vi "Log Error.vi"(10 "Log Packet":T1, 11 "Application Log in":refnum<class "Application Logger.lvclass">) -> (0 "error out":errorcluster, 3 "Application Log out":refnum<class "Application Logger.lvclass">)   [LabVIEW 2017, in "Composed Log.lvlib" / "Application Logger.lvclass"]
uses:
  <vilib>/gpm_packages/@cs/event-logger/Source/Composed Log/Application Logger/Application Logger.lvclass
  <vilib>/gpm_packages/@cs/event-logger/Source/Composed Log/Types/Log Packet.ctl
  <vilib>/gpm_packages/@cs/event-logger/Source/Composed Log/Types/Log Level.ctl
  <vilib>/gpm_packages/@cs/event-logger/Source/Composed Log/Composed Log.lvlib
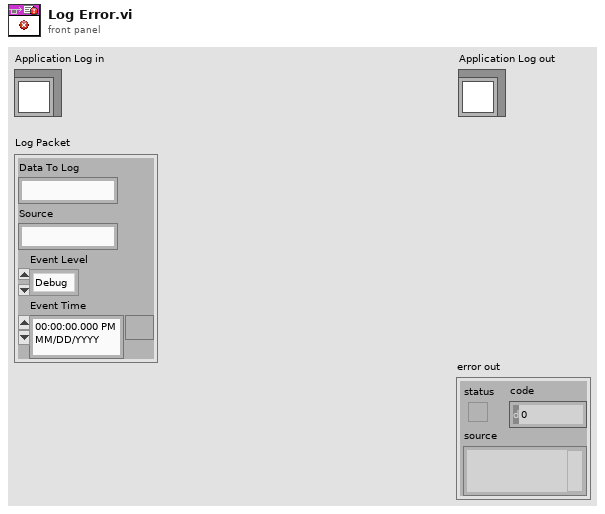
[diagram p1: front panel]
types:
  T1 = typedef "Composed Log.lvlib/Log Packet.ctl" = cluster{"Data To Log":string, "Source":string, "Event Level":T2, "Event Time":timestamp}
  T2 = typedef "Composed Log.lvlib/Log Level.ctl" = enum16{"Debug", "Info", "Warning", "Error", "Critical"}
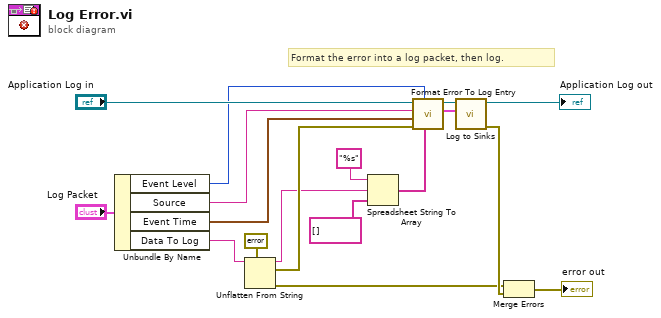
[diagram p0: block diagram]
diagram:
  # "Format the error into a log packet, then log."
  n1 = Unbundle By Name("Log Packet") -> ("Event Level"=w6:T2, "Source"=w7:string, "Event Time"=w8:timestamp, "Data To Log"=w11:string)
  n2 = Unflatten From String(type=errorcluster {"status"=FALSE, "code"=0, "source"=""} ("Error To Log"), binary string=w11) -> (rest of the binary string=w4:string, value=w9:errorcluster, error out=w5:errorcluster)  [unwired: 3 in]
  n3 = Spreadsheet String To Array(format string="%s", spreadsheet string=w4, array type (2D Dbl)=string[] [] ("rest of the binary string")) -> (array=w2:string[])  [unwired: 1 in]
  n4 = call-dynamic "Format Error To Log Entry.vi"("Error Call Chain"=w2, "Event Level"=w6, "Error To Log"=w9, "Event Time"=w8, "Error SourceID"=w7, "Application Logger In"="Application Log in") -> ("Log Packet"=w17:T1, "Application Logger out"=w15:refnum<class "Application Logger.lvclass">)  [unwired: 4 in]
  n5 = call-dynamic "Log to Sinks.vi"("Log Packet"=w17, "Asynchronous Application Log in"=w15) -> ("error out"=w13:errorcluster, "Asynchronous Application Log out"=→"Application Log out":refnum<class "Application Logger.lvclass">)  [unwired: 8 in]
  n6 = Merge Errors(w5, w13) -> (→"error out":errorcluster)
